vi "Load Overlapping Transactions.vi"(8 "error in (no error)":errorcluster, 10 "Proposed Transactions":refnum<class "Statement.lvclass">, 11 "Database in":refnum<class "Database.lvclass">) -> (0 "error out":errorcluster, 2 "Existing Transactions":refnum<class "Statement.lvclass">, 3 "Database out":refnum<class "Database.lvclass">)   [LabVIEW 2018, in "Database.lvclass"]
uses:
  Database.lvclass
  Statement/Statement.lvclass
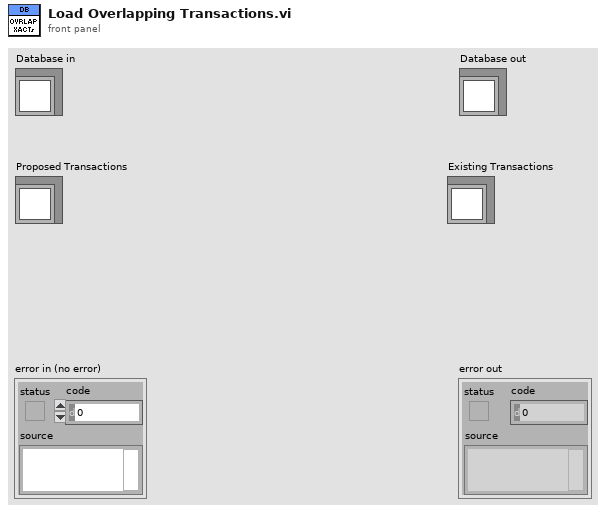
[diagram p1: front panel]
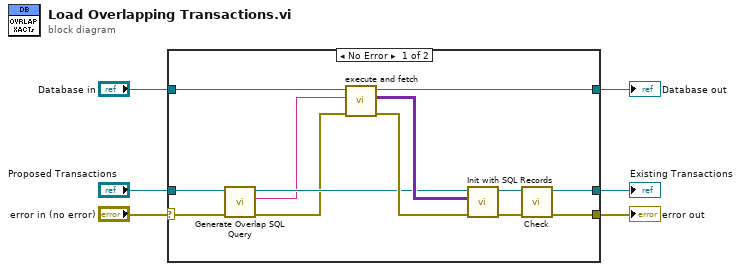
[diagram p0: block diagram]
diagram:
  n1 = case shown="No Error" "error in (no error)" {
    selector: "error in (no error)" -> [w7 w21]
    tunnel: "Proposed Transactions" -> [w12 w20]
    tunnel: [w11 w20] -> w5
    tunnel: "Database in" -> [w10 w22]
    tunnel: [w9 w21] -> w3
    tunnel: [w8 w22] -> w2
    frame No Error {
      n2 = call-dynamic "Generate Overlap SQL Query.vi"("error in (no error)"=w7, "Importing Transactions"=w12) -> ("error out"=w13:errorcluster, "Overlap Query"=w14:string, "Overlapping Records"=w15:refnum<class "Statement.lvclass">)  [unwired: 7 in]
      n3 = call "execute and fetch.vi"("error in (no error)"=w13, "SQL query"=w14, "Database in"=w10) -> ("error out"=w16:errorcluster, "recordset data"=w17:variant[][], "Database out"=w8:refnum<class "Database.lvclass">)  [unwired: 5 in, 1 out]
      n4 = call-dynamic "Init with SQL Records.vi"("error in (no error)"=w16, "SQL Dataset"=w17, "Statement in"=w15) -> ("error out"=w19:errorcluster, "Statement out"=w18:refnum<class "Statement.lvclass">)  [unwired: 7 in]
      n5 = call-dynamic "Check.vi"("error in (no error)"=w19, "Statement in"=w18) -> ("error out"=w9:errorcluster, "Statement out"=w11:refnum<class "Statement.lvclass">)  [unwired: 8 in]
    }
    frame Error {
    }
  }
  "error out" <- w3
  "Database out" <- w2
  "Existing Transactions" <- w5
